vi "Configure Multi Eval Meas List Segment Additional PUSCH Allocation.vi"(0 "VISA resource name":refnum<visa-resource-name>, 1 "Allocation (1)":T1=1, 2 "CDM Groups (1)":i32=1, 3 "Antenna Port (0)":i32, 5 "Instance (1)":T4=1, 7 "Segment (1)":T3=1, 9 "Carrier Component (1)":T2=1, 11 "error in (no error)":errorcluster, 12 "DMRS Length (1)":i32=1, 13 "DMRS Power (0.0)":dbl format="%^.3e") -> (4 "VISA resource name out":refnum<visa-resource-name>, 15 "error out":errorcluster)   [LabVIEW 2020, in "Rohde&Schwarz CMXP NR FR2 Measurement.lvlib"]
doc: "Configures special PUSCH settings, for carrier <cc>, allocation <a> in segment <no>.\n\nAttribute:\nRSCMXPNRFR2M_ATTR_MULTI_EVAL_MEASUREMENT_LIST_SEGMENT_ADDITIONAL_PUSCH_ALLOCATION\n\nRemote-control command:\nCONFigure:NRMMw:MEAS<i>:LIST:SEGMent<no>[:CC<cc>]:ALLocation<a>:PUSCh:ADDitional"
uses:
  <instrlib>/Rohde&Schwarz CMXP NR FR2 Measurement/Rohde&Schwarz CMXP NR FR2 Measurement.lvlib
  <instrlib>/Rohde&Schwarz CMXP NR FR2 Measurement/Private/_Instance.ctl
  <instrlib>/Rohde&Schwarz CMXP NR FR2 Measurement/Private/_Segment.ctl
  <instrlib>/Rohde&Schwarz CMXP NR FR2 Measurement/Private/_Carrier Component.ctl
  <instrlib>/Rohde&Schwarz CMXP NR FR2 Measurement/Private/_Allocation.ctl
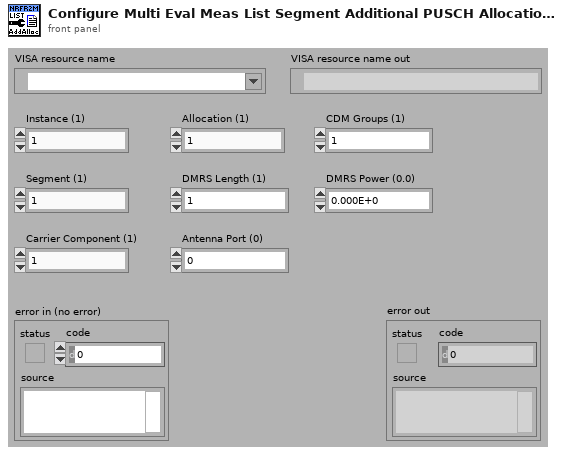
[diagram p1: front panel]
types:
  T1 = typedef "Rohde&Schwarz CMXP NR FR2 Measurement.lvlib/_Allocation.ctl" = i32
  T2 = typedef "Rohde&Schwarz CMXP NR FR2 Measurement.lvlib/_Carrier Component.ctl" = i32
  T3 = typedef "Rohde&Schwarz CMXP NR FR2 Measurement.lvlib/_Segment.ctl" = i32
  T4 = typedef "Rohde&Schwarz CMXP NR FR2 Measurement.lvlib/_Instance.ctl" = i32
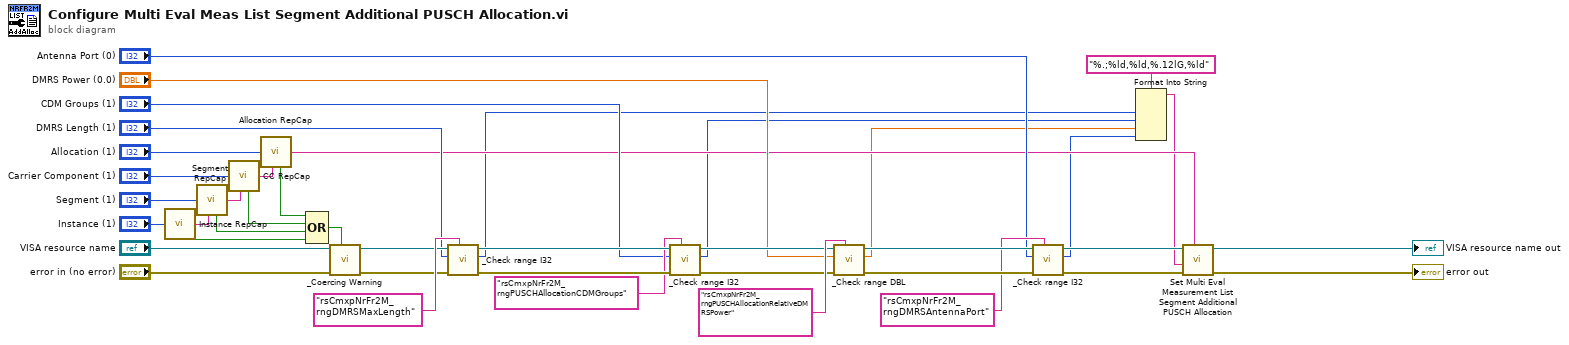
[diagram p0: block diagram]
diagram:
  n1 = call <instrlib>:"Instance RepCap.vi"("Instance In"="Instance (1)") -> ("In Range?"=w36:bool, "RepCap Identifier Out"=w2:string)  [unwired: 1 in]
  n2 = call <instrlib>:"Segment RepCap.vi"("Segment In"="Segment (1)", "RepCap String In (\"\")"=w2) -> ("In Range?"=w35:bool, "RepCap Identifier Out"=w34:string)
  n3 = call <instrlib>:"CC RepCap.vi"("CC In"="Carrier Component (1)", "RepCap String In (\"\")"=w34) -> ("In Range?"=w33:bool, "RepCap Identifier Out"=w32:string)
  n4 = call <instrlib>:"Allocation RepCap.vi"("Allocation In"="Allocation (1)", "RepCap String In (\"\")"=w32) -> ("In Range?"=w31:bool, "RepCap Identifier Out"=w9:string)
  n5 = Compound Arithmetic op=OR(w31, w33, w35, w36) -> (w38:bool)
  n6 = call <instrlib>:"_Coercing Warning.vi"("In Range?"=w38, "error in (no error)"="error in (no error)", "VISA resource name"="VISA resource name") -> ("error out"=w19:errorcluster, "VISA resource name out"=w18:refnum<visa-resource-name>)  [unwired: 7 in]
  n7 = call <instrlib>:"_Check range I32.vi"("Range Table Identifier"="rsCmxpNrFr2M_rngDMRSMaxLength", "error in (no error)"=w19, "I32 Value In"="DMRS Length (1)", "VISA resource name"=w18) -> ("error out"=w30:errorcluster, "I32 Value Out"=w7:i32, "VISA resource name out"=w29:refnum<visa-resource-name>)  [unwired: 5 in]
  n8 = call <instrlib>:"_Check range I32.vi"("Range Table Identifier"="rsCmxpNrFr2M_rngPUSCHAllocationCDMGroups", "error in (no error)"=w30, "I32 Value In"="CDM Groups (1)", "VISA resource name"=w29) -> ("error out"=w26:errorcluster, "I32 Value Out"=w6:i32, "VISA resource name out"=w25:refnum<visa-resource-name>)  [unwired: 5 in]
  n9 = call <instrlib>:"_Check range DBL.vi"("Range Table Identifier"="rsCmxpNrFr2M_rngPUSCHAllocationRelativeDMRSPower", "error in (no error)"=w26, "DBL Value In"="DMRS Power (0.0)", "VISA resource name"=w25) -> ("error out"=w23:errorcluster, "DBL Value Out"=w5:dbl, "VISA resource name out"=w24:refnum<visa-resource-name>)  [unwired: 5 in]
  n10 = call <instrlib>:"_Check range I32.vi"("Range Table Identifier"="rsCmxpNrFr2M_rngDMRSAntennaPort", "error in (no error)"=w23, "I32 Value In"="Antenna Port (0)", "VISA resource name"=w24) -> ("error out"=w12:errorcluster, "I32 Value Out"=w4:i32, "VISA resource name out"=w13:refnum<visa-resource-name>)  [unwired: 5 in]
  n11 = Format Into String(format string="%.;%ld,%ld,%.12lG,%ld", w7, w6, w5, w4) -> (resulting string=w1:string)  [unwired: 2 in, 1 out]
  n12 = call "Set Multi Eval Measurement List Segment Additional PUSCH Allocation"("Repeated Capabilities"=w9, "error in (no error)"=w12, "Multi Eval Measurement List Segment Additional PUSCH Allocation ()"=w1, "instrument handle"=w13) -> ("error out"=→"error out":errorcluster, "instrument handle out"=→"VISA resource name out":refnum<visa-resource-name>)  [unwired: 6 in]
